vi "ReadLog.vi"(8 "Error In":errorcluster, 11 "Log File Path":path) -> (0 "Error Out":errorcluster, 2 "MFC Plots":cluster{timestamp[], "Y Data":dbl[]}[](array[cluster]), 3 "Heater Plots":cluster{timestamp[], "Y Data":dbl[]}[](array[cluster]))   [LabVIEW 2012]
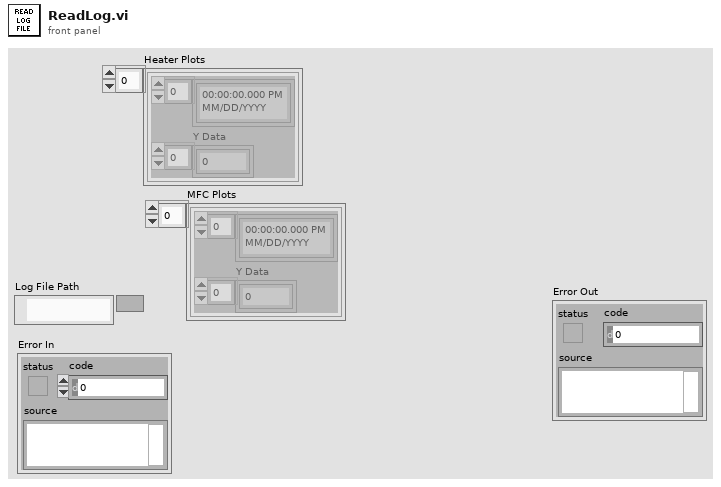
[diagram p1: front panel]
types:
  T1 = enum16{"open", "replace", "create", "open or create", "replace or create", "replace or create with confirmation"}
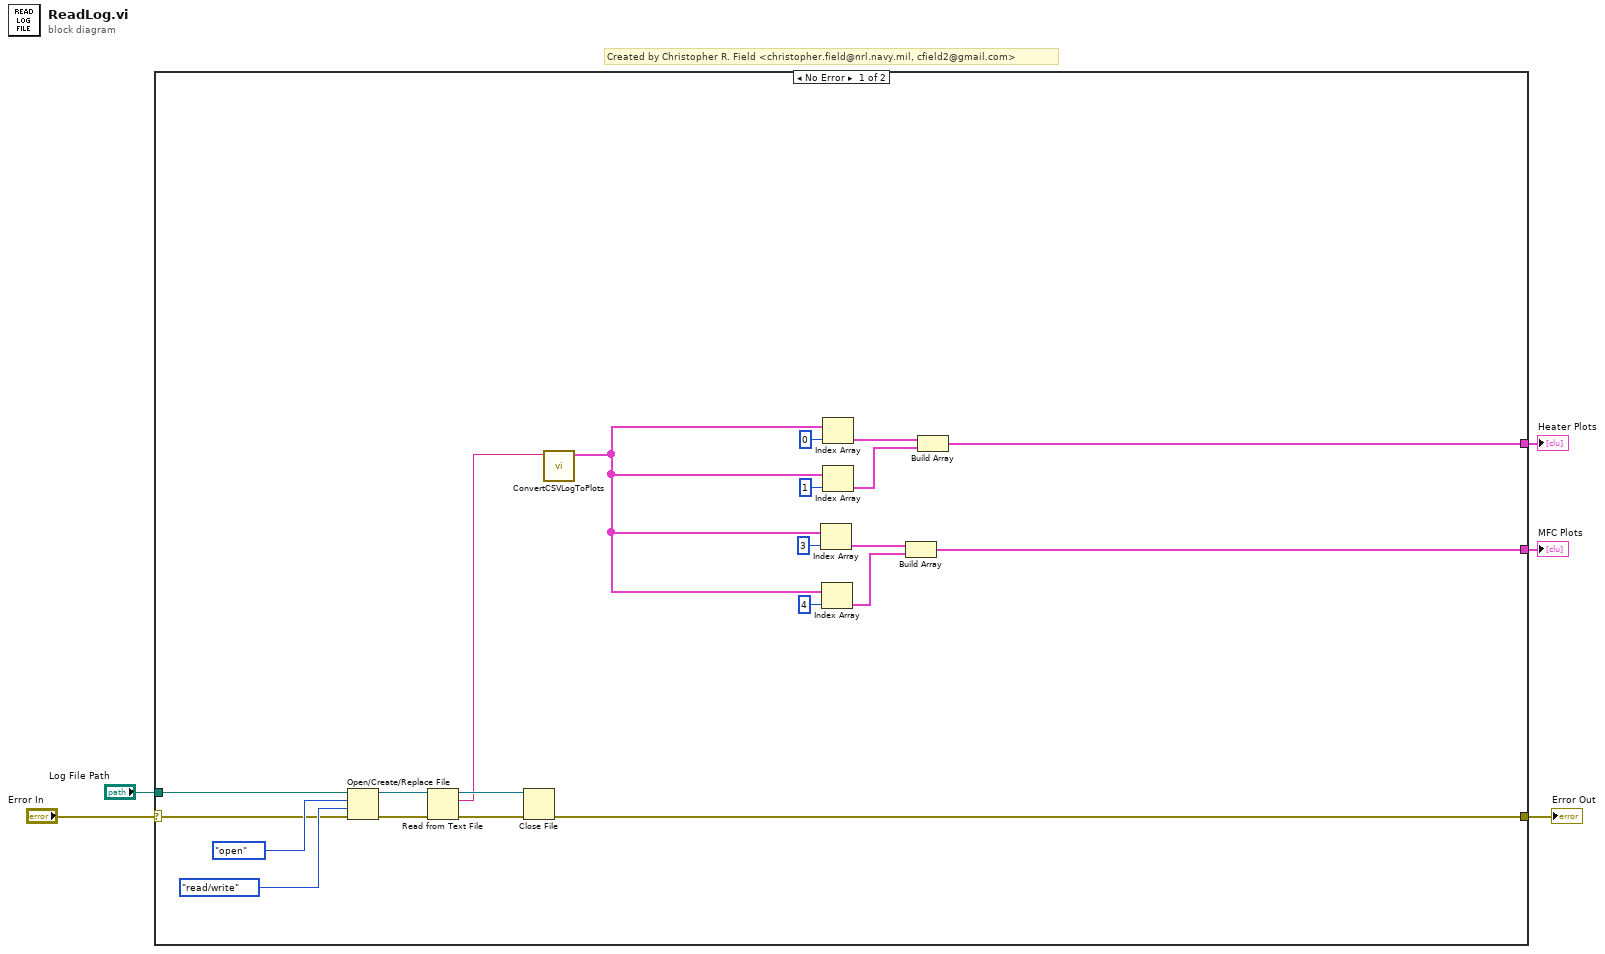
[diagram p0: block diagram]
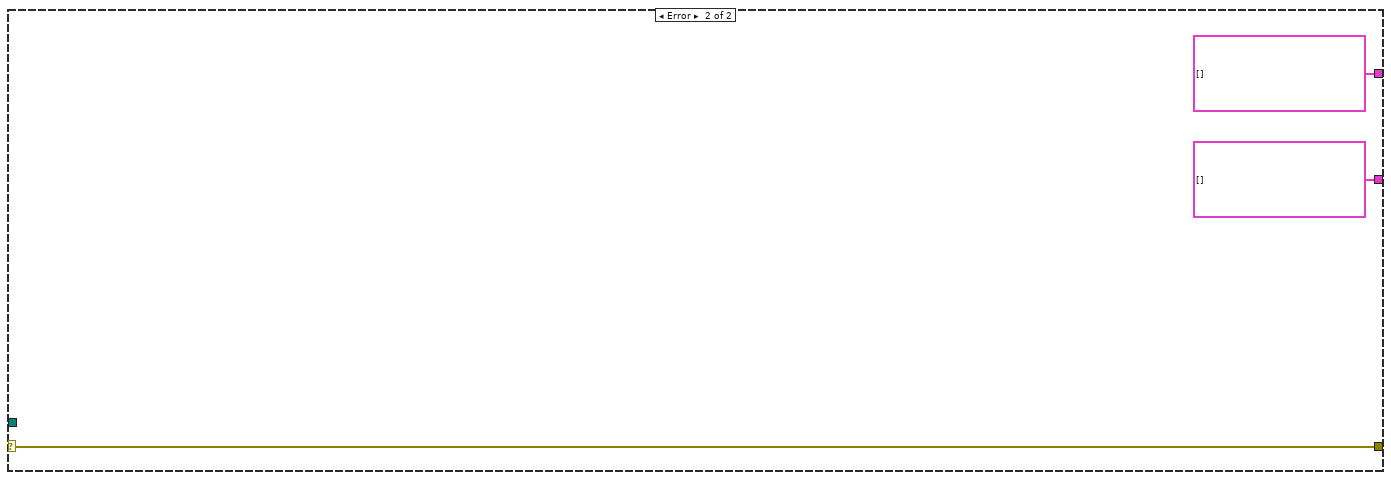
[diagram p2: hidden frame]
diagram:
  # "Created by Christopher R. Field <christopher.field@nrl.navy.mil, cfield2@gmail.com>"
  n1 = case shown="No Error" "Error In" {
    selector: "Error In" -> [w18 w29]
    tunnel: "Log File Path" -> [w26 _]
    tunnel: [w19 w29] -> w4
    tunnel: [w7 cluster{timestamp[], "Y Data":dbl[]}[] []] -> w2
    tunnel: [w6 cluster{timestamp[], "Y Data":dbl[]}[] []] -> w1
    frame No Error {
      n2 = Open/Create/Replace File(file path (use dialog)=w26, error in=w18, operation (0:open)=T1."open", access (0:read/write)=enum16{"read/write", "read-only", "write-only"}."read/write") -> (refnum out=w23:refnum<file>, error out=w22:errorcluster)  [unwired: 2 in, 1 out]
      n3 = Read from Text File(file (use dialog)=w23, error in=w22) -> (refnum out=w21:refnum<file>, text=w17:string, error out=w20:errorcluster)  [unwired: 2 in, 1 out]
      n4 = Close File(refnum=w21, error in=w20) -> (error out=w19:errorcluster)  [unwired: 1 out]
      n5 = call "ConvertCSVLogToPlots.vi"("CSV String"=w17) -> ("Plots"=w8:cluster{timestamp[], "Y Data":dbl[]}[])  [unwired: 10 in]
      n6 = Index Array(array=w8, index=3) -> (element=w10:cluster{timestamp[], "Y Data":dbl[]})
      n7 = Index Array(array=w8, index=4) -> (element=w9:cluster{timestamp[], "Y Data":dbl[]})
      n8 = Index Array(array=w8, index=0) -> (element=w12:cluster{timestamp[], "Y Data":dbl[]})
      n9 = Index Array(array=w8, index=1) -> (element=w11:cluster{timestamp[], "Y Data":dbl[]})
      n10 = Build Array(w10, w9) -> (w6:cluster{timestamp[], "Y Data":dbl[]}[])
      n11 = Build Array(w12, w11) -> (w7:cluster{timestamp[], "Y Data":dbl[]}[])
    }
    frame Error {
    }
  }
  "Error Out" <- w4
  "Heater Plots" <- w2
  "MFC Plots" <- w1
